vi "PSAE_VCH_Register Popup.vi"(7 "PopUp Name":string, 8 "Error In (no error)":errorcluster, 11 "Tree Ref":refnum<vi>) -> (0 "Error Out":errorcluster)   [LabVIEW 2016]
uses:
  ToolKit/Popup/Private/Ctrls/POP_Popup Call Parameters.ctl
  ToolKit/Popup/Private/Ctrls/POP_Data Type.ctl
  <vilib>/Utility/miscctls.llb/LVBrowseOptionsTypeDef.ctl
panel:
  # "Data Out"
  # "Data In"
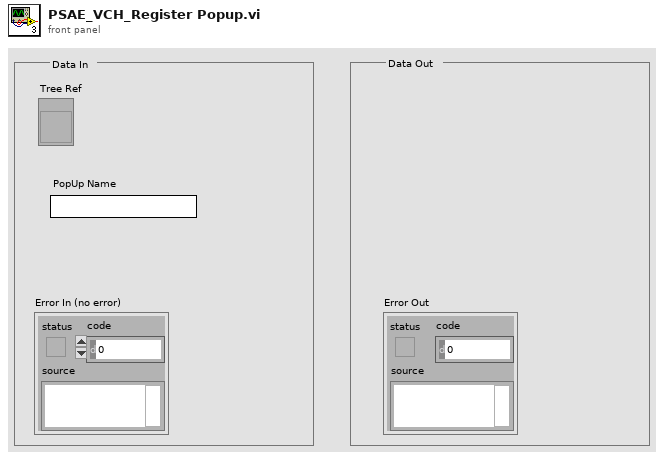
[diagram p1: front panel]
types:
  T1 = typedef "POP_Popup Call Parameters.ctl" = cluster{"Prop Type":T2, "Initial Value":variant, "Caption Strings":string[], "Ring Strings":string[], "Cell Rect":cluster{"left":i16, "top":i16, "right":i16, "bottom":i16}, "Mouse Coords":cluster{"x":i16, "y":i16}, "Call Data":variant, "Ring Values":ext[], "Browse Options":T3, "Combo Box":cluster{"Allow Undefined Strings":bool}}
  T2 = typedef "POP_Data Type.ctl" = enum16{"NO POPUP", "Unkown", "String", "Integer", "Float", "Color", "Boolean", "Ring", "Captioned String", "Captioned Integer", "Button Color", "2 Int Cluster", "4 Int Cluster", "6-Dbl Cluster", "Path", "Combox", "Time", "ShotCut String"}
  T3 = typedef "LVBrowseOptionsTypeDef.ctl" = cluster{"Prompt":string, "Match Pattern":string, "Mode":enum32{"existing file", "new file", "new or existing file", "existing dir", "new dir", "new or existing dir", "existing file (use LLBs)", "new file (use LLBs)", "new or existing file (use LLBs)", "new or existing file or directory (use LLBs)", "existing dir (use LLBs)", "new dir (use LLBs)", "new or existing dir (use LLBs)", "existing file or dir", "new file or dir", "new or existing file or dir", "existing file or dir (use LLBs)", "new file or dir (use LLBs)"}, "Start Path":path, "Pattern Label":string, "Button Text":string}
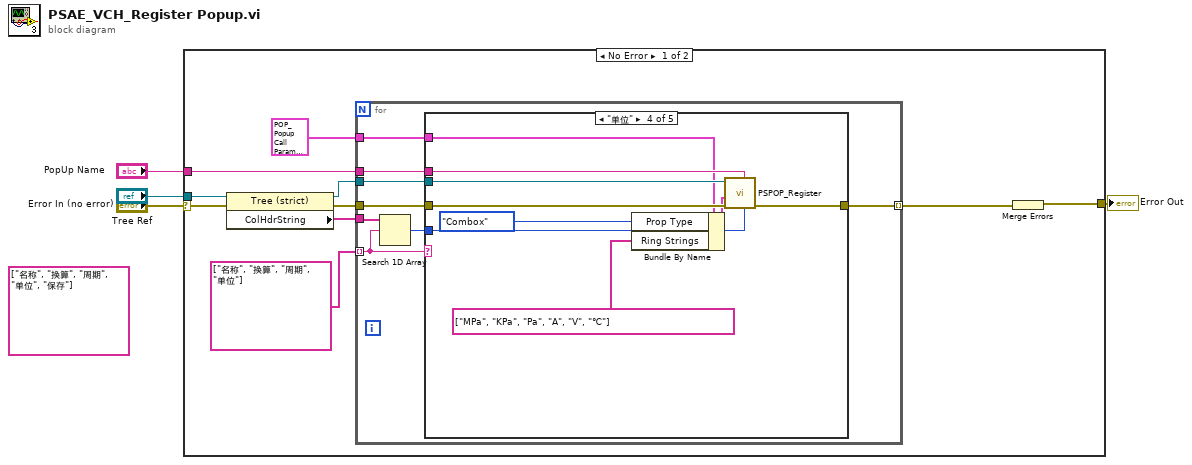
[diagram p0: block diagram]
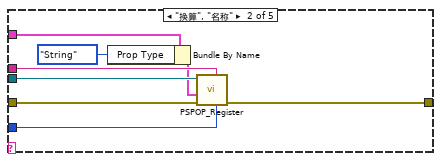
[diagram p3: hidden frame]
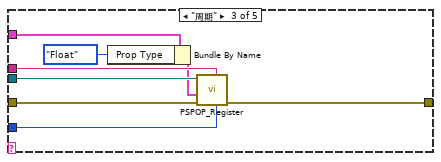
[diagram p4: hidden frame]
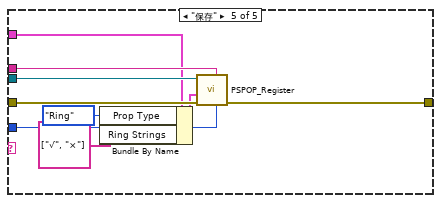
[diagram p5: hidden frame]
diagram:
  (unwired) string[] ["名称", "换算", "周期", "单位", "保存"] ("Column Header Strings[]")
  n1 = case shown="No Error" "Error In (no error)" {
    selector: "Error In (no error)" -> [w6 w58]
    tunnel: "PopUp Name" -> [w14 _]
    tunnel: "Tree Ref" -> [w13 _]
    tunnel: [w5 w58] -> w1
    frame No Error {
      n2 = property class="Tree (strict)"(reference=w13, error in=w6) -> (reference out=w7:refnum<vi>, error out=w8:errorcluster, "ColHdrString"=w10:string[])
      n3 = for {
        tunnel: w8 -> [w22]
        tunnel: w7 -> [w21]
        tunnel: w14 -> [w20]
        tunnel: [w19] -> w11 mode=indexing
        tunnel: T1 {"Prop Type"=enum."String", "Initial Value"=variant, "Caption Strings"=[], "Ring Strings"=[], "Cell Rect"={"left"=0, "top"=0, "right"=0, "bottom"=0}, "Mouse Coords"={"x"=0, "y"=0}, "Call Data"=variant, "Ring Values"=[], "Browse Options"={"Prompt"="", "Match Pattern"="", "Mode"=enum."existing file", "Start Path"=path "", "Pattern Label"="", "Button Text"=""}, "Combo Box"={"Allow Undefined Strings"=FALSE}} ("Parameters") -> [w18]
        tunnel: w10 -> [w17]
        tunnel: string[] ["名称", "换算", "周期", "单位"] ("Column Header Strings[]") -> [w16] mode=indexing
        n4 = Search 1D Array(1D array=w17, element=w16) -> (index of element=w15:i32)  [unwired: 1 in]
        n5 = case shown="\"单位\"" w16 {
          tunnel: w22 -> [w23 w31 w39 w48 w57]
          tunnel: w21 -> [_ w30 w38 w47 w56]
          tunnel: w20 -> [_ w29 w37 w46 w55]
          tunnel: [w23 w28 w36 w45 w54] -> w19
          tunnel: w18 -> [_ w27 w35 w44 w53]
          tunnel: w15 -> [_ w25 w33 w42 w51]
          frame Default {
          }
          frame "换算", "名称" {
            n6 = Bundle By Name(cluster=w27, "Prop Type"=POP_Data_Type."String") -> (w26:T1)
            n7 = call "PSPOP_Register.vi"("Col (unwired = all columns)"=w25, "Name"=w29, "error in (no error)"=w31, "Parameters"=w26, "Ctl Refnum"=w30) -> ("error out"=w28:errorcluster)  [unwired: 5 in, 1 out]
          }
          frame "周期" {
            n8 = Bundle By Name(cluster=w35, "Prop Type"=POP_Data_Type."Float") -> (w34:T1)
            n9 = call "PSPOP_Register.vi"("Col (unwired = all columns)"=w33, "Name"=w37, "error in (no error)"=w39, "Parameters"=w34, "Ctl Refnum"=w38) -> ("error out"=w36:errorcluster)  [unwired: 5 in, 1 out]
          }
          frame "单位" {
            n10 = Bundle By Name(cluster=w44, "Prop Type"=POP_Data_Type."Combox", "Ring Strings"=string[] ["MPa", "KPa", "Pa", "A", "V", "℃"]) -> (w43:T1)
            n11 = call "PSPOP_Register.vi"("Col (unwired = all columns)"=w42, "Name"=w46, "error in (no error)"=w48, "Parameters"=w43, "Ctl Refnum"=w47) -> ("error out"=w45:errorcluster)  [unwired: 5 in, 1 out]
          }
          frame "保存" {
            n12 = Bundle By Name(cluster=w53, "Prop Type"=POP_Data_Type."Ring", "Ring Strings"=string[] ["√", "×"]) -> (w52:T1)
            n13 = call "PSPOP_Register.vi"("Col (unwired = all columns)"=w51, "Name"=w55, "error in (no error)"=w57, "Parameters"=w52, "Ctl Refnum"=w56) -> ("error out"=w54:errorcluster)  [unwired: 5 in, 1 out]
          }
        }
      }
      n14 = Merge Errors(w11) -> (w5:errorcluster)
    }
    frame Error {
    }
  }
  "Error Out" <- w1
